vi "Upload.vi"(4 "attributes":refnum<class "File Attributes.lvclass">, 6 "timeout (ms)":i32=30000, 8 "error in":errorcluster, 9 "remote path":string, 10 "session in":refnum<class "Session.lvclass">, 11 "NI_SFTP.lvlib:Generic Upload Controller.lvclass":refnum<class "Generic Upload Controller.lvclass">) -> (0 "error out":errorcluster, 2 "session out":refnum<class "Session.lvclass">, 3 "NI_SFTP.lvlib:Generic Upload Controller.lvclass 2":refnum<class "Generic Upload Controller.lvclass">)   [LabVIEW 2020, in "NI_SFTP.lvlib" / "Generic Upload Controller.lvclass"]
doc: "Creates a new remote file, initialized with a byte array."
uses:
  <vilib>/net/SFTP/API/Support/Upload/Generic/Generic Upload Controller.lvclass
  <vilib>/net/SFTP/Session/Session.lvclass
  <vilib>/net/SFTP/File Attributes/File Attributes.lvclass
  <vilib>/net/SFTP/File Attributes/File Attributes.lvclass/File Attributes.ctl
  <vilib>/net/SFTP/API/Support/Command/SSH_FXP_OPEN/Input.ctl
  <vilib>/net/SFTP/API/Support/Open Flags.ctl
  <vilib>/net/SFTP/API/Support/File Attributes.ctl
  <vilib>/net/SFTP/Session/Session.lvclass/Session.ctl
  <vilib>/net/SFTP/API/Support/Command/SSH_FXP_WRITE/Input.ctl
  <vilib>/net/SFTP/Session/Handle.ctl
  <vilib>/net/SFTP/Session/Read fsync.vi
  <vilib>/net/SFTP/Session/Read block size.vi
  <vilib>/net/SFTP/API/Support/Command/SSH_FXP_CLOSE/SSH_FXP_CLOSE.lvclass
  <vilib>/net/SFTP/API/Support/Command/SSH_FXP_OPEN/SSH_FXP_OPEN.lvclass
  <vilib>/net/SFTP/API/Support/Command/SSH_FXP_WRITE/SSH_FXP_WRITE.lvclass
  <vilib>/Utility/Deadline/NI_Deadline.lvlib
  <vilib>/net/SFTP/NI_SFTP.lvlib
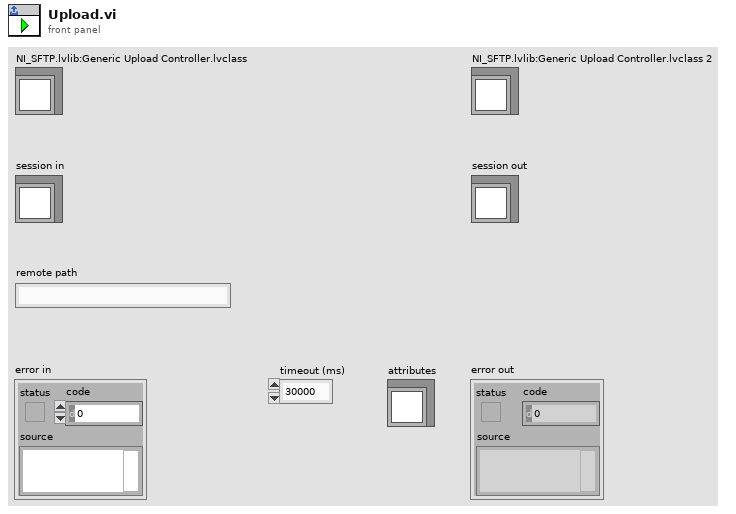
[diagram p1: front panel]
types:
  T1 = typedef "NI_SFTP.lvlib/SSH_FXP_OPEN.lvclass/Input.ctl" = cluster{"filename":string, "open flags":T2, "file attributes":T3}
  T2 = typedef "NI_SFTP.lvlib/SSH_FXP_OPEN.lvclass/Open Flags.ctl" = cluster{"SSH_FXF_READ":bool, "SSH_FXF_WRITE":bool, "SSH_FXF_APPEND":bool, "SSH_FXF_CREAT":bool, "SSH_FXF_TRUNC":bool, "SSH_FXF_EXCL":bool}
  T3 = typedef "NI_SFTP.lvlib/File Attributes.ctl" = cluster{"SSH_FILEXFER_ATTR_SIZE":bool, "size":u64, "SSH_FILEXFER_ATTR_UIDGID":bool, "uid":u32, "gid":u32, "SSH_FILEXFER_ATTR_PERMISSIONS":bool, "permissions":u32, "SSH_FILEXFER_ATTR_ACMODTIME":bool, "atime":u32, "mtime":u32, "extended":map{string, string}}
  T4 = typedef "NI_SFTP.lvlib/SSH_FXP_WRITE.lvclass/Input.ctl" = cluster{"handle":T5, "offset":u64, "data":u8[]}
  T5 = typedef "NI_SFTP.lvlib/Session.lvclass/Handle.ctl" = u8[]
  T6 = typedef "NI_Deadline.lvlib/Deadline.ctl" = cluster{"mode":T7, "deadline (ms)":u32}
  T7 = typedef "NI_Deadline.lvlib/Mode.ctl" = enum16{"Relative", "Use deadline", "Wait forever", "Nonblocking", "N/A"}
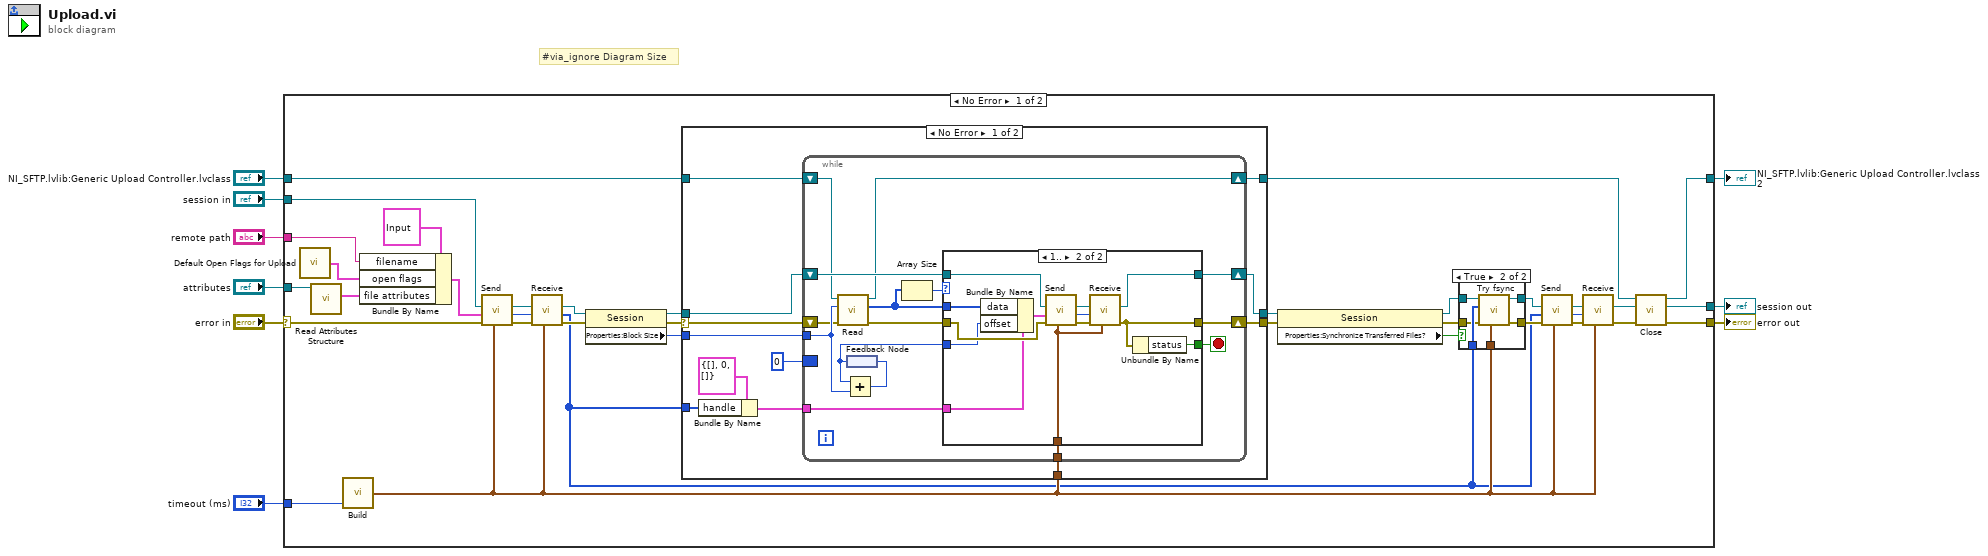
[diagram p0: block diagram]
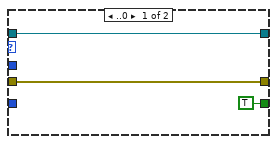
[diagram p3: hidden frame]
diagram:
  # "#via_ignore Diagram Size"
  n1 = case shown="No Error" "error in" {
    selector: "error in" -> [w39 w100]
    tunnel: "session in" -> [w27 w101]
    tunnel: "remote path" -> [w25 _]
    tunnel: [w16 w101] -> w7
    tunnel: [w10 w100] -> w6
    tunnel: "timeout (ms)" -> [w40 _]
    tunnel: "attributes" -> [w38 _]
    tunnel: "NI_SFTP.lvlib:Generic Upload Controller.lvclass" -> [w15 w99]
    tunnel: [w13 w99] -> w1
    frame No Error {
      n2 = call <vilib>:"Default Open Flags for Upload.vi"() -> ("open flags"=w24:T2)
      n3 = call <vilib>:"Read Attributes Structure.vi"("file attributes in"=w38) -> ("file attributes"=w21:T3)  [unwired: 9 in, 1 out]
      n4 = call <vilib>:"Build.vi"("timeout (ms)"=w40) -> ("Deadline out"=w36:T6)  [unwired: 2 in]
      n5 = Bundle By Name(cluster=T1 {"filename"="", "open flags"={"SSH_FXF_READ"=FALSE, "SSH_FXF_WRITE"=FALSE, "SSH_FXF_APPEND"=FALSE, "SSH_FXF_CREAT"=FALSE, "SSH_FXF_TRUNC"=FALSE, "SSH_FXF_EXCL"=FALSE}, "file attributes"={"SSH_FILEXFER_ATTR_SIZE"=FALSE, "size"=0, "SSH_FILEXFER_ATTR_UIDGID"=FALSE, "uid"=0, "gid"=0, "SSH_FILEXFER_ATTR_PERMISSIONS"=FALSE, "permissions"=0, "SSH_FILEXFER_ATTR_ACMODTIME"=FALSE, "atime"=0, "mtime"=0, "extended"={}}} ("input"), "filename"=w25, "open flags"=w24, "file attributes"=w21) -> (w23:T1)
      n6 = call <vilib>:"Send.vi"("deadline"=w36, "error in"=w39, "input"=w23, "session in"=w27) -> ("error out"=w44:errorcluster, "request id"=w22:u32, "session out"=w43:refnum<class "Session.lvclass">)  [unwired: 4 in, 1 out]
      n7 = call <vilib>:"Receive.vi"("deadline"=w36, "error in"=w44, "request id"=w22, "session in"=w43) -> ("error out"=w34:errorcluster, "handle"=w19:T5, "session out"=w20:refnum<class "Session.lvclass">)  [unwired: 4 in, 1 out]
      n8 = property on="Property Node" class="Session"(reference=w20, error in=w34) -> (reference out=w35:refnum<class "Session.lvclass">, error out=w33:errorcluster, "Properties:Block Size"=w32:i32)
      n9 = case shown="No Error" w33 {
        selector: w33 -> [w59 w97]
        tunnel: w35 -> [w60 w98]
        tunnel: [w63 w98] -> w31
        tunnel: w19 -> [w55 _]
        tunnel: [w62 w97] -> w12
        tunnel: w36 -> [w61 _]
        tunnel: w32 -> [w58 _]
        tunnel: w15 -> [w57 w96]
        tunnel: [w53 w96] -> w14
        frame No Error {
          n10 = Bundle By Name(cluster=T4 {"handle"=[], "offset"=0, "data"=[]} ("input"), "handle"=w55) -> (w54:T4)
          n11 = while {
            shift-right: [w76] -> w62
            shift-left: w59 -> [w69]
            shift-right: [w78] -> w63
            shift-left: w60 -> [w72]
            border: u64 0 ("len") -> [_]
            tunnel: w61 -> [w73]
            tunnel: w58 -> [w70]
            shift-right: [w67] -> w53
            shift-left: w57 -> [w71]
            tunnel: w54 -> [w65]
            stop <- w74 stop-if-true
            n12 = call-dynamic "Read.vi"("error in (no error)"=w69, "count"=w70, "Generic Upload Controller in"=w71) -> ("error out"=w68:errorcluster, "data"=w66:u8[], "Generic Upload Controller out"=w67:refnum<class "Generic Upload Controller.lvclass">)  [unwired: 6 in]
            n13 = feedback #1() -> (w77:u64)
            n14 = Add(x=w77, y=w70) -> (x+y=w79:u64)
            n15 = feedback-in #1(w79) -> ()
            n16 = Array Size(array=w66) -> (size(s)=w75:i32)
            n17 = case shown="1.." w75 {
              tunnel: w72 -> [w82 w95]
              tunnel: w68 -> [w81 w94]
              tunnel: [w82 w90] -> w78
              tunnel: w77 -> [_ w84]
              tunnel: w66 -> [_ w85]
              tunnel: [w81 w89] -> w76
              tunnel: [TRUE ("status") w88] -> w74
              tunnel: w73 -> [_ w87]
              tunnel: w65 -> [_ w86]
              frame ..0 {
              }
              frame 1.. {
                n18 = Bundle By Name(cluster=w86, "data"=w85, "offset"=w84) -> (w83:T4)
                n19 = call <vilib>:"Send.vi"("deadline"=w87, "error in"=w94, "input"=w83, "session in"=w95) -> ("error out"=w91:errorcluster, "request id"=w92:u32, "session out"=w93:refnum<class "Session.lvclass">)  [unwired: 4 in, 1 out]
                n20 = call <vilib>:"Receive.vi"("deadline"=w87, "error in"=w91, "request id"=w92, "session in"=w93) -> ("error out"=w89:errorcluster, "session out"=w90:refnum<class "Session.lvclass">)  [unwired: 4 in, 2 out]
                n21 = Unbundle By Name(w89) -> ("status"=w88:bool)
              }
            }
          }
        }
        frame Error {
        }
      }
      n22 = property on="Property Node" class="Session"(reference=w31, error in=w12) -> (reference out=w30:refnum<class "Session.lvclass">, error out=w29:errorcluster, "Properties:Synchronize Transferred Files?"=w28:bool)
      n23 = case shown="True" w28 {
        tunnel: [w46 w52] -> w18
        tunnel: [w45 w51] -> w37
        tunnel: w19 -> [_ w50]
        tunnel: w36 -> [_ w49]
        tunnel: w30 -> [w46 w48]
        tunnel: w29 -> [w45 w47]
        frame False {
        }
        frame True {
          n24 = call <vilib>:"Try fsync.vi"("Deadline in"=w49, "error in (no error)"=w47, "handle"=w50, "session in"=w48) -> ("error out"=w51:errorcluster, "session out"=w52:refnum<class "Session.lvclass">)  [unwired: 6 in]
        }
      }
      n25 = call <vilib>:"Send.vi"("deadline"=w36, "error in"=w37, "handle"=w19, "session in"=w18) -> ("error out"=w42:errorcluster, "request id"=w17:u32, "session out"=w41:refnum<class "Session.lvclass">)  [unwired: 4 in, 1 out]
      n26 = call <vilib>:"Receive.vi"("deadline"=w36, "error in"=w42, "request id"=w17, "session in"=w41) -> ("error out"=w11:errorcluster, "session out"=w16:refnum<class "Session.lvclass">)  [unwired: 4 in, 2 out]
      n27 = call-dynamic "Close.vi"("error in (no error)"=w11, "Generic Upload Controller in"=w14) -> ("error out"=w10:errorcluster, "Generic Upload Controller out"=w13:refnum<class "Generic Upload Controller.lvclass">)  [unwired: 8 in]
    }
    frame Error {
    }
  }
  "error out" <- w6
  "session out" <- w7
  "NI_SFTP.lvlib:Generic Upload Controller.lvclass 2" <- w1
